vi "2_Speed_Gearbox_AutoShifter.vi"(8 "PhoenixMotorControlDevRef 2":T1={"DeviceStatus"={"status"=FALSE, "code"=0, "source"=""}, "Type"=enum."PWM", "PWM"={"PWM Channel"=enum."Invalid", "DeadBand"={"Name"="", "maxPositivePwm"=0, "minPositivePwm"=0, "centerPwm"=0, "maxNegativePwm"=0, "minNegativePwm"=0, "angularRange"=0}}, "CAN"={"Device Number"=0, "SetOutput VI Ref"=variant(enum8{"Percent VBus", "Current", "Speed", "Position", "Voltage"} enum."Percent VBus"), "GetOutput VI Ref"=variant(refnum<k1> refnum), "Enable VI Ref"=variant(dbl 12.0), "Disable VI Ref"=variant(enum8{"Percent VBus", "Speed", "Position", "Slave", "Unchanged / Invalid", "Voltage Compensation", "Current", "Motion Profile"} enum."Percent VBus"), "Data"=variant}, "Invert"=FALSE, "DIO PWM"={"PWM \"Enable\" Channel"=enum."Invalid", "DIOChannel"=enum."Invalid", "PWM Rate"=0.0}}, 11 "PhoenixMotorControlDevRef":T1={"DeviceStatus"={"status"=FALSE, "code"=0, "source"=""}, "Type"=enum."PWM", "PWM"={"PWM Channel"=enum."Invalid", "DeadBand"={"Name"="", "maxPositivePwm"=0, "minPositivePwm"=0, "centerPwm"=0, "maxNegativePwm"=0, "minNegativePwm"=0, "angularRange"=0}}, "CAN"={"Device Number"=0, "SetOutput VI Ref"=variant(enum8{"Percent VBus", "Current", "Speed", "Position", "Voltage"} enum."Percent VBus"), "GetOutput VI Ref"=variant(refnum<k1> refnum), "Enable VI Ref"=variant(dbl 12.0), "Disable VI Ref"=variant(enum8{"Percent VBus", "Speed", "Position", "Slave", "Unchanged / Invalid", "Voltage Compensation", "Current", "Motion Profile"} enum."Percent VBus"), "Data"=variant}, "Invert"=FALSE, "DIO PWM"={"PWM \"Enable\" Channel"=enum."Invalid", "DIOChannel"=enum."Invalid", "PWM Rate"=0.0}}) -> ()   [LabVIEW 2017]
uses:
  <vilib>/Rock Robotics/WPI/MotorControl/WPI_MotorControlDeviceRef.ctl
  <vilib>/Rock Robotics/WPI/MotorControl/WPI_MotorControlType.ctl
  <vilib>/Rock Robotics/SystemInterfaces/DIO/FPGA_DIOPWMChannel.ctl
  <vilib>/Rock Robotics/WPI/PWM/WPI_PWMDeadband.ctl
  <vilib>/Rock Robotics/SystemInterfaces/DIO/FPGA_DIOChannel.ctl
  <vilib>/Rock Robotics/WPI/Solenoid/WPI_SolenoidValue.ctl
  <vilib>/Rock Robotics/WPI/ThirdParty/Phoenix-LabVIEW/Motor Controller/Get/CTRE_Phoenix_MotorController_GetQuadratureData.vi
  <vilib>/Rock Robotics/WPI/Solenoid/WPI_SolenoidSetEnum.vi
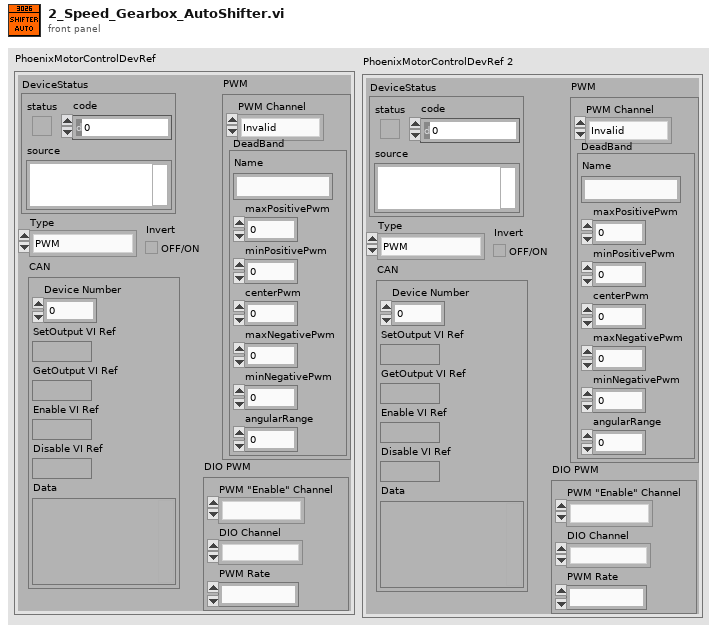
[diagram p1: front panel]
types:
  T1 = typedef "WPI_MotorControlDeviceRef.ctl" = cluster{"DeviceStatus":errorcluster, "Type":T2, "PWM":cluster{"PWM Channel":T3, "DeadBand":T4}, "CAN":cluster{"Device Number":u8, "SetOutput VI Ref":variant, "GetOutput VI Ref":variant, "Enable VI Ref":variant, "Disable VI Ref":variant, "Data":variant}, "Invert":bool, "DIO PWM":cluster{"PWM \"Enable\" Channel":T3, "DIOChannel":T5, "PWM Rate":dbl}}
  T2 = typedef "WPI_MotorControlType.ctl" = enum16{"PWM", "CAN", "DIO PWM"}
  T3 = typedef "FPGA_DIOPWMChannel.ctl" = enum8{"PWM 0", "PWM 1", "PWM 2", "PWM 3", "PWM 4", "PWM 5", "PWM 6", "PWM 7", "PWM 8", "PWM 9", "PWM MXP 0", "PWM MXP 1", "PWM MXP 2", "PWM MXP 3", "PWM MXP 4", "PWM MXP 5", "PWM MXP 6", "PWM MXP 7", "PWM MXP 8", "PWM MXP 9", "Invalid"}
  T4 = typedef "WPI_PWMDeadband.ctl" = cluster{"Name":string, "maxPositivePwm":i32, "minPositivePwm":i32, "centerPwm":i32, "maxNegativePwm":i32, "minNegativePwm":i32, "angularRange":u16}
  T5 = typedef "FPGA_DIOChannel.ctl" = enum8{"DIO 0", "DIO 1", "DIO 2", "DIO 3", "DIO 4", "DIO 5", "DIO 6", "DIO 7", "DIO 8", "DIO 9", "DIO MXP 0", "DIO MXP 1", "DIO MXP 2", "DIO MXP 3", "DIO MXP 4", "DIO MXP 5", "DIO MXP 6", "DIO MXP 7", "DIO MXP 8", "DIO MXP 9", "DIO MXP 10", "DIO MXP 11", "DIO MXP 12", "DIO MXP 13", "DIO MXP 14", "DIO MXP 15", "SPI Port CS1", "SPI Port CS2", "SPI Port CS3", "SPI Port MISO", "SPI Port MOSI", "Invalid"}
  T6 = typedef "WPI_SolenoidValue.ctl" = enum16{"Off", "On", "Forward", "Reverse"}
  T7 = typedef "WPI_SolenoidDevRef.ctl" = cluster{"DevStatus":errorcluster, "Pneumatics Control Module":u8, "Forward Solenoid Channel":T8, "Reverse Solenoid Channel":T8}
  T8 = typedef "WPI_SolenoidChannel.ctl" = enum8{"Solenoid 0", "Solenoid 1", "Solenoid 2", "Solenoid 3", "Solenoid 4", "Solenoid 5", "Solenoid 6", "Solenoid 7", "Invalid"}
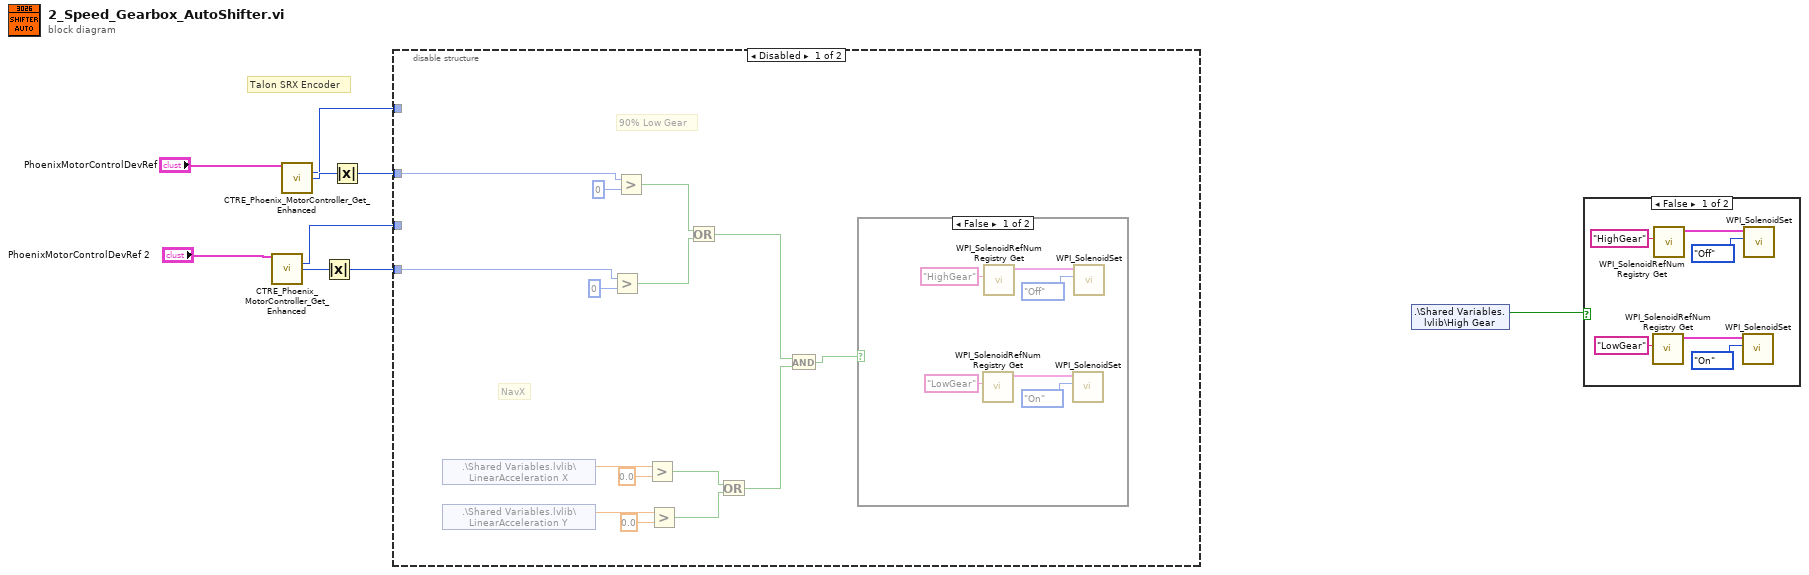
[diagram p0: block diagram]
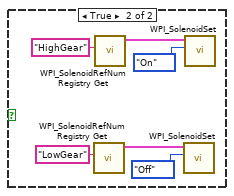
[diagram p2: hidden frame]
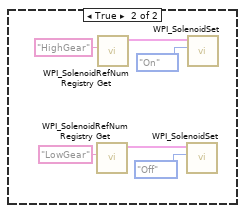
[diagram p3: hidden frame]
diagram:
  # "Talon SRX Encoder"
  n1 = call-poly <vilib>:"CTRE_Phoenix_MotorController_Get_Enhanced.vi"("PhoenixMotorControlDevRef"="PhoenixMotorControlDevRef 2") -> ("Quadrature Position"=w1:i32, "Quadrature Velocity"=w4:i32)  [unwired: 11 in, 2 out]
  n2 = call-poly <vilib>:"CTRE_Phoenix_MotorController_Get_Enhanced.vi"("PhoenixMotorControlDevRef"="PhoenixMotorControlDevRef") -> ("Quadrature Position"=w2:i32, "Quadrature Velocity"=w5:i32)  [unwired: 11 in, 2 out]
  n3 = Absolute Value(x=w4) -> (abs(x)=w3:i32)
  n4 = Absolute Value(x=w5) -> (abs(x)=w6:i32)
  n5 = disable-structure shown="Disabled" {
    disable-tunnel: w6 -> [w11 _]
    disable-tunnel: w3 -> [w10 _]
    disable-tunnel: w2 -> [_ _]
    disable-tunnel: w1 -> [_ _]
    frame Disabled {
      # "NavX"
      # "90% Low Gear"
      n6 = shared-variable ".\\Shared Variables.lvlib\\LinearAcceleration X"() -> (w21:dbl)  [unwired: 1 in, 1 out]
      n7 = shared-variable ".\\Shared Variables.lvlib\\LinearAcceleration Y"() -> (w22:dbl)  [unwired: 1 in, 1 out]
      n8 = Greater?(x=w10, y=0) -> (0:w23:bool)
      n9 = Greater?(x=w11, y=0) -> (0:w24:bool)
      n10 = Greater?(x=w21, y=0.0) -> (0:w20:bool)
      n11 = Greater?(x=w22, y=0.0) -> (0:w19:bool)
      n12 = Or(x=w24, y=w23) -> (x .or. y?=w18:bool)
      n13 = Or(x=w20, y=w19) -> (x .or. y?=w17:bool)
      n14 = And(x=w18, y=w17) -> (x .and. y?=w16:bool)
      n15 = case shown="False" w16 {
        frame False {
          n16 = call <vilib>:"WPI_SolenoidRefNum Registry Get.vi"("refnum name"="LowGear") -> ("SolenoidDevRef"=w28:T7)  [unwired: 9 in, 1 out]
          n17 = call <vilib>:"WPI_SolenoidRefNum Registry Get.vi"("refnum name"="HighGear") -> ("SolenoidDevRef"=w30:T7)  [unwired: 9 in, 1 out]
          n18 = call-poly <vilib>:"WPI_SolenoidSet.vi"("Value"=WPI_SolenoidValue."On", "SolenoidDevRef"=w28) -> ()  [unwired: 8 in, 2 out]
          n19 = call-poly <vilib>:"WPI_SolenoidSet.vi"("Value"=WPI_SolenoidValue."Off", "SolenoidDevRef"=w30) -> ()  [unwired: 8 in, 2 out]
        }
        frame True {
          n20 = call <vilib>:"WPI_SolenoidRefNum Registry Get.vi"("refnum name"="LowGear") -> ("SolenoidDevRef"=w34:T7)  [unwired: 9 in, 1 out]
          n21 = call <vilib>:"WPI_SolenoidRefNum Registry Get.vi"("refnum name"="HighGear") -> ("SolenoidDevRef"=w36:T7)  [unwired: 9 in, 1 out]
          n22 = call-poly <vilib>:"WPI_SolenoidSet.vi"("Value"=WPI_SolenoidValue."Off", "SolenoidDevRef"=w34) -> ()  [unwired: 8 in, 2 out]
          n23 = call-poly <vilib>:"WPI_SolenoidSet.vi"("Value"=WPI_SolenoidValue."On", "SolenoidDevRef"=w36) -> ()  [unwired: 8 in, 2 out]
        }
      }
    }
    frame Enabled {
    }
  }
  n24 = shared-variable ".\\Shared Variables.lvlib\\High Gear"() -> (w9:bool)  [unwired: 1 in, 1 out]
  n25 = case shown="False" w9 {
    frame False {
      n26 = call <vilib>:"WPI_SolenoidRefNum Registry Get.vi"("refnum name"="LowGear") -> ("SolenoidDevRef"=w40:T7)  [unwired: 9 in, 1 out]
      n27 = call <vilib>:"WPI_SolenoidRefNum Registry Get.vi"("refnum name"="HighGear") -> ("SolenoidDevRef"=w42:T7)  [unwired: 9 in, 1 out]
      n28 = call-poly <vilib>:"WPI_SolenoidSet.vi"("Value"=WPI_SolenoidValue."On", "SolenoidDevRef"=w40) -> ()  [unwired: 8 in, 2 out]
      n29 = call-poly <vilib>:"WPI_SolenoidSet.vi"("Value"=WPI_SolenoidValue."Off", "SolenoidDevRef"=w42) -> ()  [unwired: 8 in, 2 out]
    }
    frame True {
      n30 = call <vilib>:"WPI_SolenoidRefNum Registry Get.vi"("refnum name"="LowGear") -> ("SolenoidDevRef"=w46:T7)  [unwired: 9 in, 1 out]
      n31 = call <vilib>:"WPI_SolenoidRefNum Registry Get.vi"("refnum name"="HighGear") -> ("SolenoidDevRef"=w48:T7)  [unwired: 9 in, 1 out]
      n32 = call-poly <vilib>:"WPI_SolenoidSet.vi"("Value"=WPI_SolenoidValue."Off", "SolenoidDevRef"=w46) -> ()  [unwired: 8 in, 2 out]
      n33 = call-poly <vilib>:"WPI_SolenoidSet.vi"("Value"=WPI_SolenoidValue."On", "SolenoidDevRef"=w48) -> ()  [unwired: 8 in, 2 out]
    }
  }
